vi "Save Specific Worksheet as CSV.vi"(8 "error in (no error)":errorcluster, 9 "Destination Directory":path, 10 "Worksheet Name":string, 11 "ExcelRefs in":T1) -> (0 "error out":errorcluster, 2 "New CSV File":path, 3 "ExcelRefs dup":T1)   [LabVIEW 2011]
uses:
  Controls/Excel Refs.ctl
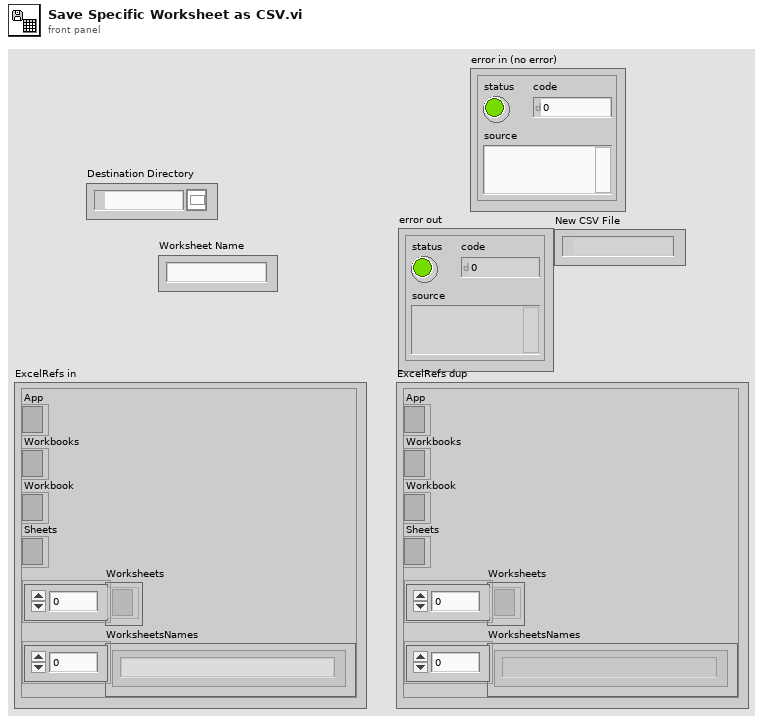
[diagram p1: front panel]
types:
  T1 = typedef "Excel Refs.ctl" = cluster{"App":refnum<k7>, "Workbooks":refnum<k7>, "Workbook":refnum<k7>, "Sheets":refnum<k7>, "Worksheets":refnum<k7>[], "WorksheetsNames":string[]}
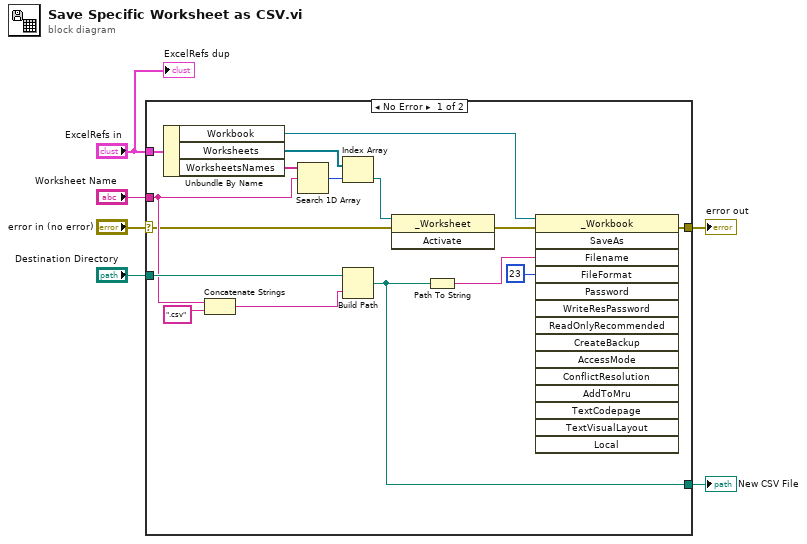
[diagram p0: block diagram]
diagram:
  n1 = case shown="No Error" "error in (no error)" {
    selector: "error in (no error)" -> [w7 w23]
    tunnel: "Destination Directory" -> [w15 _]
    tunnel: "Worksheet Name" -> [w14 _]
    tunnel: [w11 _] -> w4
    tunnel: [w9 w23] -> w3
    tunnel: "ExcelRefs in" -> [w8 _]
    frame No Error {
      n2 = Unbundle By Name(w8) -> ("Workbook"=w18:refnum<k7>, "Worksheets"=w21:refnum<k7>[], "WorksheetsNames"=w22:string[])
      n3 = Concatenate Strings(w14, ".csv" ("string")) -> (w12:string)
      n4 = Search 1D Array(1D array=w22, element=w14) -> (index of element=w17:i32)  [unwired: 1 in]
      n5 = Index Array(array=w21, index=w17) -> (element=w20:refnum<k7>)
      n6 = Build Path(base path=w15, name or relative path=w12) -> (appended path=w11:path)
      n7 = invoke class="_Worksheet" method="Activate"(reference=w20, error in=w7) -> (error out=w16:errorcluster)  [unwired: 1 in, 2 out]
      n8 = Path To String(path=w11) -> (string=w10:string)
      n9 = invoke class="_Workbook" method="SaveAs"(reference=w18, error in=w16, "Filename"=w10, "FileFormat"=23) -> (error out=w9:errorcluster)  [unwired: 11 in, 14 out]
    }
    frame Error {
    }
  }
  "error out" <- w3
  "New CSV File" <- w4
  "ExcelRefs dup" <- "ExcelRefs in"
